vi "Initialize TCP.vi"(8 "error in":errorcluster, 11 "Telnet V2 in":refnum<class "Telnet V2.lvclass">) -> (0 "error out":errorcluster, 3 "Telnet V2 out":refnum<class "Telnet V2.lvclass">)   [LabVIEW 2018, in "Telnet V2.lvlib" / "Telnet V2.lvclass"]
uses:
  Telnet V2.lvclass
  C:/AME Test Engineering/LabVIEW/PPLs/LiDAR/Parent/LiDAR.lvlibp/LiDAR.lvclass
  Telnet V2.lvclass/Telnet V2.ctl
  PPLs/Configuration/Configuration.lvlibp/Configuration.lvclass
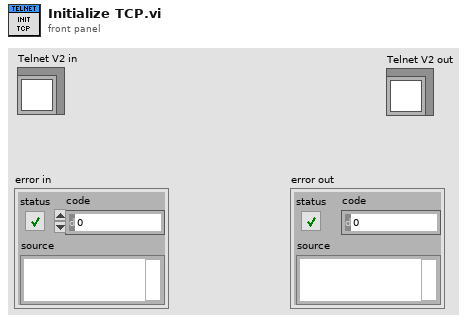
[diagram p1: front panel]
types:
  T1 = cluster{"Configuration":refnum<class "Configuration.lvclass">, "Network":cluster{"TCP":cluster{"IP Address":string, "Port":u16}, "UDP":cluster{"IP Address":string, "Port":u16}}, "Azimuth":cluster{"Min >=-60":string, "Max <=+60":string}, "Elevation":cluster{"FOV":string, "Offset":string, "Scan Pattern":enum16{"Triangle", "Snap"}, "Frequency":string}, "Data Algo":enum16{"Resim", "Point Cloud"}}
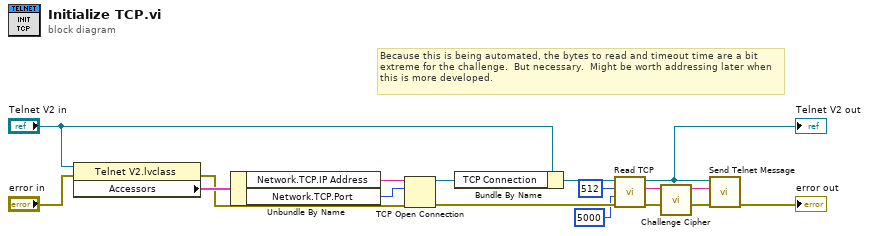
[diagram p0: block diagram]
diagram:
  # "Because this is being automated, the bytes to read and timeout time are a bit extreme for the challenge.  But necessary.  Might be worth addressing later when this is more developed."
  n1 = property class="Telnet V2.lvclass"(reference="Telnet V2 in", error in="error in") -> (error out=w8:errorcluster, "Accessors"=w12:T1)  [unwired: 1 out]
  n2 = Unbundle By Name(w12) -> ("Network.TCP.IP Address"=w14:string, "Network.TCP.Port"=w13:u16)
  n3 = TCP Open Connection(address=w14, remote port or service name=w13, error in (no error)=w8) -> (connection ID=w10:refnum<k5>, error out=w5:errorcluster)  [unwired: 2 in]
  n4 = Bundle By Name(cluster="Telnet V2 in", "TCP Connection"=w10) -> (w7:refnum<class "Telnet V2.lvclass">)
  n5 = call-dynamic "Read TCP.vi"("error in (no error)"=w5, "Timeout (ms)"=5000, "Bytes to Read"=512, "Telnet V2 in"=w7) -> ("error out"=w4:errorcluster, "Data Out"=w3:string, "Telnet V2 out"=w6:refnum<class "Telnet V2.lvclass">)  [unwired: 5 in]
  "Telnet V2 out" <- w6
  n6 = call "Challenge Cipher.vi"("Message In"=w3) -> ("Response"=w15:string)  [unwired: 10 in]
  n7 = call "Send Telnet Message.vi"("error in"=w4, "Message In"=w15, "Telnet V2 in"=w6) -> ("error out"=→"error out":errorcluster)  [unwired: 8 in]
